vi "DIAdem Open Reference.vi"(8 "error in (no error)":errorcluster, 10 "Show Environment (F)":bool) -> (0 "error out":errorcluster, 3 "DIAdem Reference":T1)   [LabVIEW 2017]
doc: "This VI opens a reference to a DIAdem application on the same computer. DIAdem must be installed. If DIAdem is not already running, it is started by the VI."
uses:
  <vilib>/ExportToExcel/DIAdem Reference.ctl
  <vilib>/ExportToExcel/Window Names.ctl
  <vilib>/ExportToExcel/Window Modes.ctl
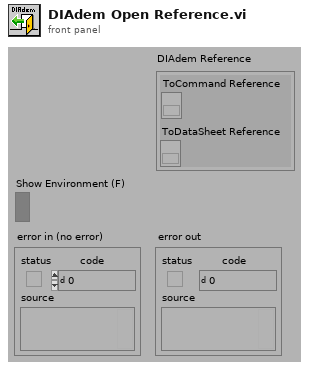
[diagram p1: front panel]
types:
  T1 = typedef "DIAdem Reference.ctl" = cluster{"ToCommand Reference":refnum<k7>, "ToDataSheet Reference":refnum<k7>}
  T2 = typedef "Window Modes.ctl" = enum16{"OPEN", "CLOSE", "SHOW", "MAXIMIZE", "MINIMIZE", "NORMAL", "FULLSIZE"}
  T3 = typedef "Window Names.ctl" = u16
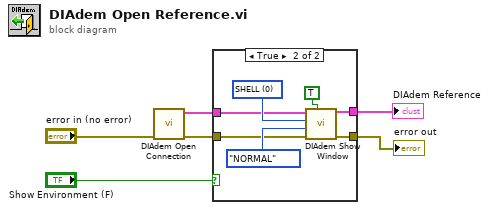
[diagram p0: block diagram]
diagram:
  n1 = call <vilib>:"DIAdem Open Connection.vi"("error in (no error)"="error in (no error)") -> ("error out"=w2:errorcluster, "DIAdem Reference"=w3:T1)  [unwired: 9 in]
  n2 = case shown="True" "Show Environment (F)" {
    tunnel: [w8 w15] -> w4
    tunnel: [w7 w14] -> w6
    tunnel: w3 -> [w8 w10]
    tunnel: w2 -> [w7 w9]
    frame False {
    }
    frame True {
      w13 = T3 0 items=["SHELL", "NAVIGATOR", "ANALYSIS", "REPORT", "VIEW", "VISUAL", "DAC"] ("window")
      n3 = call <vilib>:"DIAdem Show Window.vi"("bring to front? (F)"=TRUE ("Bring to Front? (F)"), "error in (no error)"=w9, "mode"=Window_Modes."NORMAL", "window"=w13, "DIAdem Reference"=w10) -> ("error out"=w14:errorcluster, "DIAdem Reference"=w15:T1)  [unwired: 5 in]
    }
  }
  "error out" <- w6
  "DIAdem Reference" <- w4
